vi "Read Adjacent Containers.vi"(7 "Exclude Source":refnum<class "Message Enqueuer.lvclass">, 8 "error in (no error)":errorcluster, 11 "Syringe Line in":refnum<class "Syringe Line.lvclass">) -> (0 "error out":errorcluster, 2 "Adjacent Containers":refnum<class "Message Enqueuer.lvclass">[](array[class]), 3 "Syringe Line out":refnum<class "Syringe Line.lvclass">)   [LabVIEW 2015, in "cRIO-Carbondioxide.lvlib" / "CO2-Actor.lvlib" / "Syringe Line.lvclass"]
uses:
  Syringe Line.lvclass
  <vilib>/ActorFramework/Message Enqueuer/Message Enqueuer.lvclass
  CO2 Actor/CO2 Actor.lvclass
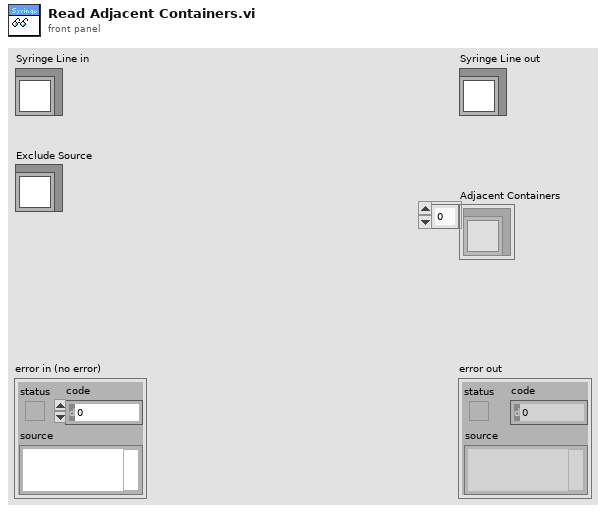
[diagram p1: front panel]
types:
  T1 = typedef "Dedicated Enqueuers.ctl" = cluster{"Freezers":cluster{"Syringe":refnum<class "Message Enqueuer.lvclass">, "Tank 1":refnum<class "Message Enqueuer.lvclass">, "Tank 2":refnum<class "Message Enqueuer.lvclass">, "Tank 3":refnum<class "Message Enqueuer.lvclass">, "Tank 4":refnum<class "Message Enqueuer.lvclass">}, "Heaters":cluster{"Syringe":refnum<class "Message Enqueuer.lvclass">, "Piston":refnum<class "Message Enqueuer.lvclass">}, "Blowers":cluster{"Tank 1":refnum<class "Message Enqueuer.lvclass">, "Tank 2":refnum<class "Message Enqueuer.lvclass">, "Tank 3":refnum<class "Message Enqueuer.lvclass">, "Tank 4":refnum<class "Message Enqueuer.lvclass">, "Syringe":refnum<class "Message Enqueuer.lvclass">}, "Sample Line":refnum<class "Message Enqueuer.lvclass">, "Storage Line":refnum<class "Message Enqueuer.lvclass">, "Transfer Line":refnum<class "Message Enqueuer.lvclass">, "Syringe Stepper":refnum<class "Message Enqueuer.lvclass">, "Syringe Line":refnum<class "Message Enqueuer.lvclass">, "Capillary Line":refnum<class "Message Enqueuer.lvclass">, "Preparation Line":refnum<class "Message Enqueuer.lvclass">, "Turbo":refnum<class "Message Enqueuer.lvclass">, "Vacuum":refnum<class "Message Enqueuer.lvclass">, "He Line":refnum<class "Message Enqueuer.lvclass">, "Cylinder":refnum<class "Message Enqueuer.lvclass">}
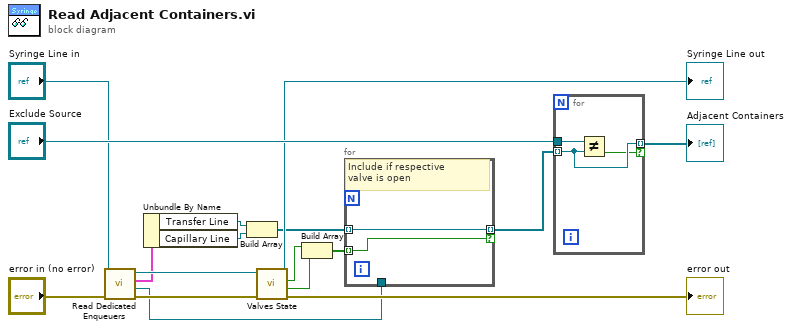
[diagram p0: block diagram]
diagram:
  n1 = call "Read Dedicated Enqueuers.vi"("error in (no error)"="error in (no error)", "CO2 Actor in"="Syringe Line in") -> ("error out"=w13:errorcluster, "DedicatedEnQrs"=w1:refnum<queue>, "Dedicated Enqueuers"=w9:T1, "CO2 Actor out"=w11:refnum<class "Syringe Line.lvclass">)  [unwired: 6 in]
  n2 = Unbundle By Name(w9) -> ("Transfer Line"=w7:refnum<class "Message Enqueuer.lvclass">, "Capillary Line"=w8:refnum<class "Message Enqueuer.lvclass">)
  n3 = Build Array(w7, w8) -> (w6:refnum<class "Message Enqueuer.lvclass">[])
  n4 = call "Valves State.vi"("error in (no error)"=w13, "Syringe in"=w11) -> ("error out"=→"error out":errorcluster, "Valve Capillar Open"=w5:bool, "Valve Transfer Line Open"=w2:bool, "Syringe out"=→"Syringe Line out":refnum<class "Syringe Line.lvclass">)  [unwired: 6 in]
  n5 = Build Array(w2, w5) -> (w4:bool[])
  n6 = for {
    tunnel: w6 -> [w19] mode=indexing
    tunnel: w4 -> [w18] mode=indexing
    tunnel: [w19] -> w3 mode=indexing if=w18
    tunnel: w1 -> [_]
    # "Include if respective\nvalve is open"
  }
  n7 = for {
    tunnel: w3 -> [w21] mode=indexing
    tunnel: "Exclude Source" -> [w22]
    tunnel: [w21] -> w16 mode=indexing if=w20
    n8 = Not Equal?(x=w22, y=w21) -> (x != y?=w20:bool)
  }
  "Adjacent Containers" <- w16
